vi "Keithley DMM7510 Buffer Fetch Slice.vi"(5 "End Index":i32, 6 "Timeout (10000 ms)":i32=10000 format="%#.6g", 7 "Start Index":i32, 8 "error in (no error)":errorcluster, 9 "Buffer Elements":u16(ring) items=["Date", "Extra", "Formatted", "Fractional", "Relative", "Seconds", "Status", "Time", "Timestamp", "Unit"], 10 "Buffer Name":string="defbuffer1", 11 "VISA resource name":refnum<visa-resource-name>) -> (0 "error out":errorcluster, 1 "Element Value":string[](array[string]), 2 "Measurements":dbl[](array[numeric]), 3 "VISA resource name out":refnum<visa-resource-name>)   [LabVIEW 2016]
uses:
  Keithley DMM7510.lvlib
panel:
  out "length":i32
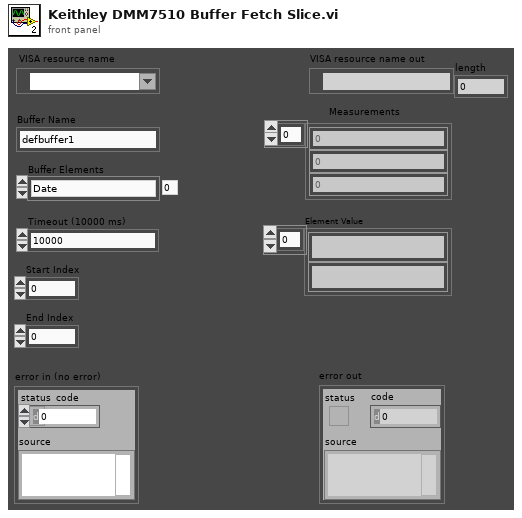
[diagram p1: front panel]
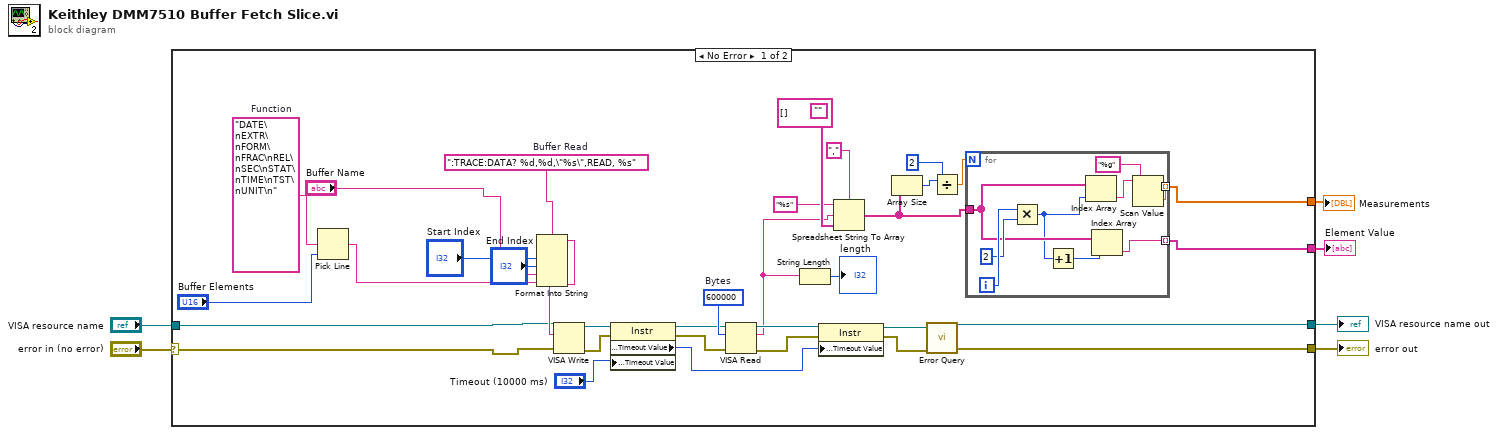
[diagram p0: block diagram]
diagram:
  n1 = case shown="No Error" "error in (no error)" {
    selector: "error in (no error)" -> [w10 w50]
    tunnel: [w39 w50] -> w6
    tunnel: [w38 w51] -> w5
    tunnel: [w16 _] -> w4
    tunnel: "VISA resource name" -> [w11 w51]
    tunnel: [w7 _] -> w1
    frame No Error {
      (unwired) ""
      w24 = "DATE\nEXTR\nFORM\nFRAC\nREL\nSEC\nSTAT\nTIME\nTST\nUNIT\n"  # Function
      w27 = ":TRACE:DATA? %d,%d,\"%s\",READ, %s"  # Buffer Read
      w40 = u32 600000  # Bytes
      n2 = Pick Line(multi-line string=w24, line index="Buffer Elements") -> (output string=w15:string)  [unwired: 1 out]
      n3 = Format Into String(format string=w27, "Start Index", "End Index", "Buffer Name", w15) -> (resulting string=w26:string)  [unwired: 2 in, 1 out]
      n4 = VISA Write(VISA resource name=w11, write buffer=w26, error in (no error)=w10) -> (VISA resource name out=w37:refnum<visa-resource-name>, error out=w36:errorcluster)  [unwired: 1 out]
      n5 = property class="Instr"(reference=w37, error in=w36, "General Settings:Timeout Value"="Timeout (10000 ms)") -> (reference out=w35:refnum<visa-resource-name>, error out=w34:errorcluster, "General Settings:Timeout Value"=w28:u32)
      n6 = VISA Read(VISA resource name=w35, byte count=w40, error in (no error)=w34) -> (VISA resource name out=w32:refnum<visa-resource-name>, read buffer=w9:string, error out=w30:errorcluster)  [unwired: 1 out]
      n7 = String Length(string=w9) -> (length=→"length":i32)
      n8 = property class="Instr"(reference=w32, error in=w30, "General Settings:Timeout Value"=w28) -> (reference out=w31:refnum<visa-resource-name>, error out=w29:errorcluster)
      n9 = Spreadsheet String To Array(delimiter (Tab)=",", format string="%s", spreadsheet string=w9, array type (2D Dbl)=string[] []) -> (array=w21:string[])
      n10 = Array Size(array=w21) -> (size(s)=w19:i32)
      n11 = call "Error Query.vi"("error in (no error)"=w29, "VISA resource name"=w31) -> ("error out"=w39:errorcluster, "VISA resource name out"=w38:refnum<visa-resource-name>)  [unwired: 6 in, 2 out]
      n12 = Divide(x=w19, y=2) -> (x/y=w17:dbl)
      n13 = for {
        N: w17 -> [_]
        tunnel: w21 -> [w47]
        tunnel: [w42] -> w7 mode=indexing
        tunnel: [w45] -> w16 mode=indexing
        i -> [w49]
        n14 = Multiply(x=w49, y=2) -> (x*y=w41:i32)
        n15 = Increment(x=w41) -> (x+1=w46:i32)
        n16 = Index Array(array=w47, index=w41) -> (element=w44:string)
        n17 = Index Array(array=w47, index=w46) -> (element=w45:string)
        n18 = Scan Value(string=w44, format string="%g") -> (value=w42:dbl)  [unwired: 1 in, 1 out]
      }
    }
    frame Error {
    }
  }
  "error out" <- w6
  "VISA resource name out" <- w5
  "Element Value" <- w4
  "Measurements" <- w1
